vi "addLink.vi"(6 "Append to End":bool, 8 "error in (no error)":errorcluster, 10 "subNode in":refnum<data-value>, 11 "superNode in":refnum<class "xceNode.lvclass">) -> (0 "error out":errorcluster, 2 "subNode out":refnum<data-value>, 3 "superNode out":refnum<class "xceNode.lvclass">)   [LabVIEW 2013, in "xceNode.lvclass"]
doc: "Adds a link between a superNode and its subNode. Used to add nodes to the tree data structure."
uses:
  xceNode.lvclass
  xceNode.lvclass/xceNode.ctl
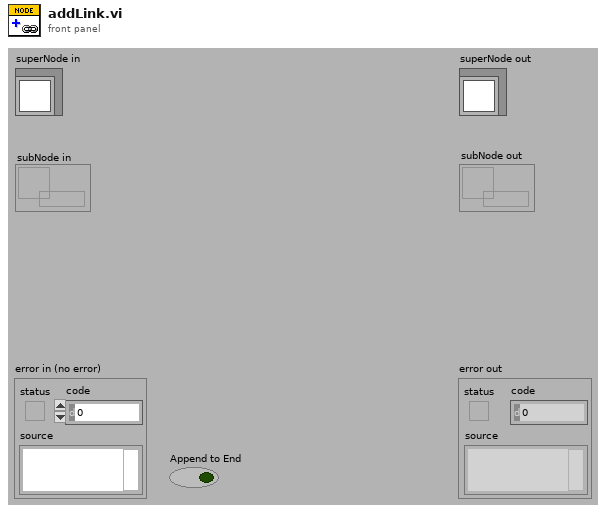
[diagram p1: front panel]
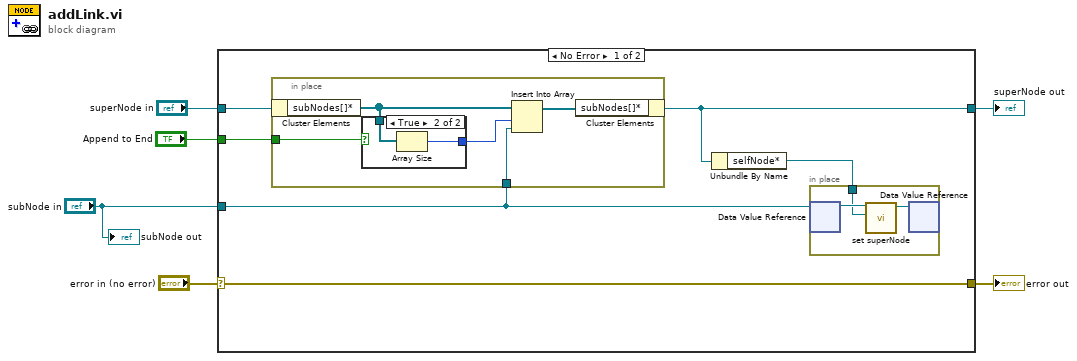
[diagram p0: block diagram]
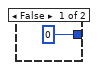
[diagram p2: hidden frame]
diagram:
  n1 = case shown="No Error" "error in (no error)" {
    selector: "error in (no error)" -> [w12 w25]
    tunnel: [w12 w25] -> w5
    tunnel: [w10 w24] -> w3
    tunnel: "superNode in" -> [w11 w24]
    tunnel: "subNode in" -> [w9 _]
    tunnel: "Append to End" -> [w7 _]
    frame No Error {
      n2 = in-place {
        in-place-border: w9 -> [w20]
        in-place-border: w7 -> [w18]
        n3 = in-place-cluster #1(w11) -> ("subNodes[]*"=w16:refnum<data-value>[])
        n4 = case shown="True" w18 {
          tunnel: [0 ("index") w22] -> w17
          tunnel: w16 -> [_ w23]
          frame False {
          }
          frame True {
            n5 = Array Size(array=w23) -> (size(s)=w22:i32)
          }
        }
        n6 = Insert Into Array(array=w16, index=w17, new element=w20) -> (w19:refnum<data-value>[])
        n7 = in-place-cluster #1("subNodes[]*"=w19) -> (w10:refnum<class "xceNode.lvclass">)
      }
      n8 = Unbundle By Name(w10) -> ("selfNode*"=w8:refnum<data-value>)
      n9 = in-place {
        in-place-border: w8 -> [w13]
        n10 = in-place-dvr #2(w9) -> (w15:refnum<class "xceNode.lvclass">)  [unwired: 1 out]
        n11 = call "set superNode.vi"("superNode*"=w13, "xceNode in"=w15) -> ("xceNode out"=w14:refnum<class "xceNode.lvclass">)  [unwired: 8 in, 1 out]
        n12 = in-place-dvr #2(w14) -> ()  [unwired: 2 out]
      }
    }
    frame Error {
    }
  }
  "error out" <- w5
  "superNode out" <- w3
  "subNode out" <- "subNode in"
